vi "Power Law Guess Parameters.vi"(10 "Y":dbl[](array[numeric]), 11 "X":dbl[](array[numeric])) -> (1 "Power Law Guess Parameters":dbl[](array[numeric]))   [LabVIEW 2021, in "Fits.lvlib"]
uses:
  Fits.lvlib
  <userlib>/_OpenG.lib/array/array.llb/Filter 1D Array (DBL)__ogtk.vi
  <userlib>/_OpenG.lib/array/array.llb/Delete Elements from 1D Array (DBL)__ogtk.vi
  <userlib>/_OpenG.lib/array/array.llb/openg_array.lvlib
  <vilib>/Analysis/NI_AALPro.lvlib
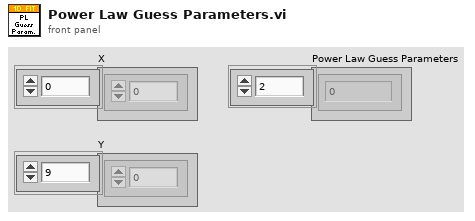
[diagram p1: front panel]
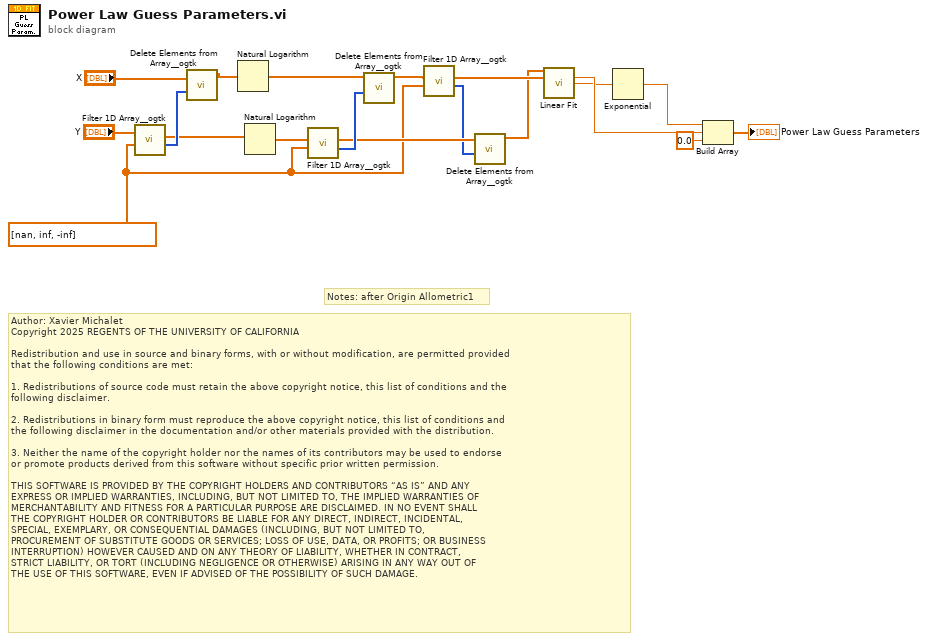
[diagram p0: block diagram]
diagram:
  w4 = dbl[] [nan, inf, -inf] ("items to filter")
  # "Author: Xavier Michalet\nCopyright 2025 REGENTS OF THE UNIVERSITY OF CALIFORNIA\n\nRedistribution and use in source and binary forms, with or without modification, are permitted provided\nthat the following conditions are met:\n\n1. Redistributions of source code must retain the above copyright notice, this list of conditions and the\nfollowing disclaimer.\n\n2. Redistributions in binary form must reproduce the above copyright notice, this list of conditions and\nthe following disclaimer in the documentation and/or other materials provided with the distribution.\n\n3. Neither the name of the copyright holder nor the names of its contributors may be used to endorse \nor promote products derived from this software without specific prior written permission.\n\nTHIS SOFTWARE IS PROVIDED BY THE COPYRIGHT HOLDERS AND CONTRIBUTORS “AS IS” AND ANY \nEXPRESS OR IMPLIED WARRANTIES, INCLUDING, BUT NOT LIMITED TO, THE IMPLIED WARRANTIES OF\nMERCHANTABILITY AND FITNESS FOR A PARTICULAR PURPOSE ARE DISCLAIMED. IN NO EVENT SHALL\nTHE COPYRIGHT HOLDER OR CONTRIBUTORS BE LIABLE FOR ANY DIRECT, INDIRECT, INCIDENTAL, \nSPECIAL, EXEMPLARY, OR CONSEQUENTIAL DAMAGES (INCLUDING, BUT NOT LIMITED TO, \nPROCUREMENT OF SUBSTITUTE GOODS OR SERVICES; LOSS OF USE, DATA, OR PROFITS; OR BUSINESS\nINTERRUPTION) HOWEVER CAUSED AND ON ANY THEORY OF LIABILITY, WHETHER IN CONTRACT, \nSTRICT LIABILITY, OR TORT (INCLUDING NEGLIGENCE OR OTHERWISE) ARISING IN ANY WAY OUT OF\nTHE USE OF THIS SOFTWARE, EVEN IF ADVISED OF THE POSSIBILITY OF SUCH DAMAGE."
  # "Notes: after Origin Allometric1"
  n1 = call-poly <userlib>:"Filter 1D Array__ogtk.vi"("items to filter"=w4, "array"="Y") -> ("filtered item indices"=w12:i32[], "filtered array"=w3:dbl[])  [unwired: 4 in]
  n2 = call-poly <userlib>:"Delete Elements from Array__ogtk.vi"("indices"=w12, "array"="X") -> ("array w/ subset deleted"=w11:dbl[])  [unwired: 8 in, 1 out]
  n3 = Natural Logarithm(1:w11) -> (0:w10:dbl[])
  n4 = Natural Logarithm(1:w3) -> (0:w18:dbl[])
  n5 = call-poly <userlib>:"Filter 1D Array__ogtk.vi"("items to filter"=w4, "array"=w18) -> ("filtered item indices"=w17:i32[], "filtered array"=w7:dbl[])  [unwired: 4 in]
  n6 = call-poly <userlib>:"Delete Elements from Array__ogtk.vi"("indices"=w17, "array"=w10) -> ("array w/ subset deleted"=w9:dbl[])  [unwired: 8 in, 1 out]
  n7 = call-poly <userlib>:"Filter 1D Array__ogtk.vi"("items to filter"=w4, "array"=w9) -> ("filtered item indices"=w6:i32[], "filtered array"=w8:dbl[])  [unwired: 4 in]
  n8 = call-poly <userlib>:"Delete Elements from Array__ogtk.vi"("indices"=w6, "array"=w7) -> ("array w/ subset deleted"=w5:dbl[])  [unwired: 8 in, 1 out]
  n9 = call <vilib>:"Linear Fit.vi"("Y"=w5, "X"=w8) -> ("slope"=w16:dbl, "intercept"=w15:dbl)  [unwired: 9 in, 3 out]
  n10 = Exponential(1:w15) -> (0:w2:dbl)
  n11 = Build Array(w2, w16, 0.0 ("element")) -> (→"Power Law Guess Parameters":dbl[])
